vi "(SubVI) ADC(read) Rate Options_YCC.vi"(4 "ADC Rate for 20bit (ms)":T1(ring)=enum."3750 Hz") -> (0 "Sampling Rate for reading (Hz)":dbl, 2 "waiting code for Reading (20bits)":dbl)   [LabVIEW 2014]
panel:
  # "3 -> 267us, 4 -> 500us , 5 -> 1ms , 6 -> 2ms, 7 -> 10ms , 8 -> 17ms , 9 -> 20ms"
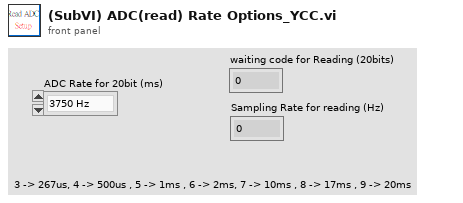
[diagram p1: front panel]
types:
  T1 = enum16{"50 Hz", "60 Hz", "100 Hz", "500 Hz", "1000 Hz", "2000 Hz", "3750 Hz"}
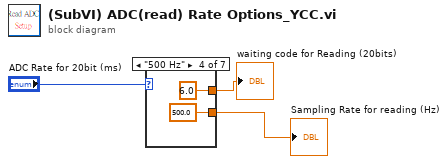
[diagram p0: block diagram]
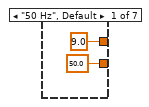
[diagram p2: hidden frame]
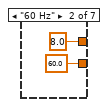
[diagram p3: hidden frame]
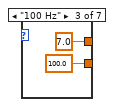
[diagram p4: hidden frame]
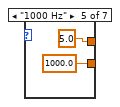
[diagram p5: hidden frame]
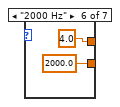
[diagram p6: hidden frame]
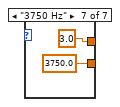
[diagram p7: hidden frame]
diagram:
  n1 = case shown="\"500 Hz\"" "ADC Rate for 20bit (ms)" {
    tunnel: [9.0 8.0 7.0 6.0 5.0 4.0 3.0] -> w1
    tunnel: [50.0 60.0 100.0 500.0 1000.0 2000.0 3750.0] -> w2
    frame "50 Hz", Default {
    }
    frame "60 Hz" {
    }
    frame "100 Hz" {
    }
    frame "500 Hz" {
    }
    frame "1000 Hz" {
    }
    frame "2000 Hz" {
    }
    frame "3750 Hz" {
    }
  }
  "Sampling Rate for reading (Hz)" <- w2
  "waiting code for Reading (20bits)" <- w1
